vi "HeadTailContinuousGWNInitialize.vi"(8 "error in (no error)":errorcluster, 11 "Stimulus in":refnum<class "HeadTailContinuousGWN.lvclass">) -> (0 "error out":errorcluster, 3 "Stimulus out":refnum<class "HeadTailContinuousGWN.lvclass">)   [LabVIEW 2019, in "HeadTailContinuousGWN.lvclass"]
uses:
  HeadTailContinuousGWN.lvclass
  StimulusObject.lvclass
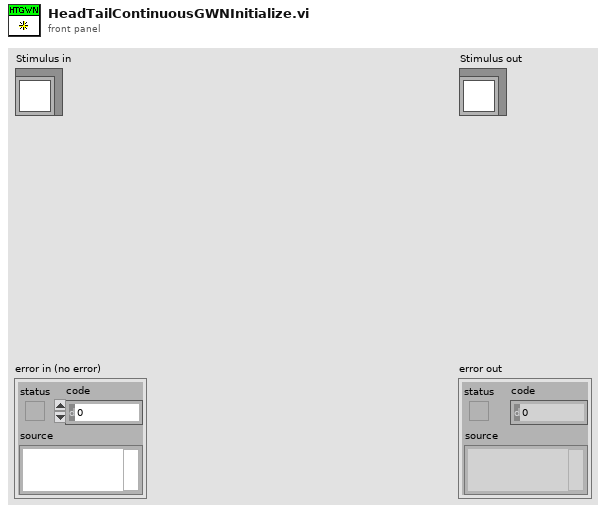
[diagram p1: front panel]
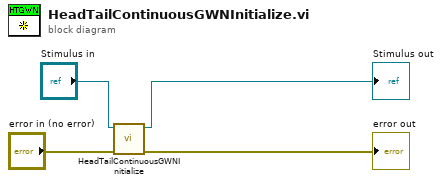
[diagram p0: block diagram]
diagram:
  n1 = call-parent "HeadTailContinuousGWNInitialize.vi"("error in (no error)"="error in (no error)", "Stimulus in"="Stimulus in") -> ("error out"=→"error out":errorcluster, "Stimulus out"=→"Stimulus out":refnum<class "HeadTailContinuousGWN.lvclass">)  [unwired: 8 in]
